vi "Main Tclk.vi"() -> ()   [LabVIEW 2018] (continued)
  T7 = cluster{"SEM Scan Parameters":cluster{"X size (um)":sgl, "Y size (um)":sgl, "X center (um)":dbl, "Y center (um)":dbl, "X size (V)":dbl, "X size auto":bool, "X stig":sgl[][], "Y stig":sgl[][], "X aln":sgl[][], "Y aln":sgl[][], "Scan rate (Hz)":u32, "Oversampling":u32, "Oversampling auto":bool, "Frame line rampdown ratio":sgl, "Pixel size (nm)":sgl, "WD (mm)":sgl[][], "X tiles":u8, "Y tiles":u8, "Overlap (um)":sgl, "Interlaced":bool, "dX (um)":sgl[], "dY (um)":sgl[], "Frames":u8}, "Detector Information":cluster{"Brightness A":dbl, "Contrast A":dbl, "Detector B name":string, "Brightness B":dbl, "Contrast B":dbl, "Detector C name":string, "Detector D name":string}, "SEM Options":cluster{"GetInfo":bool, "Set Det A para":bool, "Set WD":bool, "Set Mag":bool, "Set stig":bool, "Set aln":bool, "Display":bool, "Save":bool, "8-bit":bool, "Detector A":bool, "Detector B":bool, "Detector C":bool, "Detector D":bool, "Inverse A":bool, "Inverse B":bool, "Inverse C":bool, "Inverse D":bool, "Inverse PNG":bool, "Freeze":bool, "PNG only":bool, "Upload":bool, "Delete after upload":bool}, "Focus Index Options":cluster{"Keep aspect ratio":bool, "Show Focus Index":bool, "Focus Index primary grid center":bool, "X Grids":u8[][], "Y Grids":u8[][], "Primary X index":u8[][], "Primary Y index":u8[][]}, "Image fit to":u8, "File Information":cluster{"File path":path, "Notes":string, "Save recipe":bool, "Load recipe":bool, "Sample ID":string}, "Low mag SEM":cluster{"Low mag scan":bool, "Prior to main scan":bool, "Low mag interval":u32, "Low mag scan FOV (micron)":dbl, "Low mag scan rate (Hz)":u32, "Show HM box":bool}, "Mid Mag SEM":cluster{"Mid mag scan":bool, "Prior to main scan":bool, "Mid mag interval":u32, "X size (um)":sgl, "Y size (um)":sgl, "X center (um)":dbl, "Y center (um)":dbl, "Mid mag scan rate (Hz)":u32, "Pixel size (nm)":dbl, "Show MM box":bool}, "FIB-SEM Angle":dbl, "Milling para":cluster{"X resolution":u32, "Z resolution":u32, "X offset (um)":sgl, "Z offset (um)":sgl, "X center (um)":sgl, "Z center (um)":sgl, "X size (um)":sgl, "Z size (um)":sgl, "UL-Ang":sgl, "UR-Ang":sgl, "Line milling time (s)":sgl, "Z-step (nm)":dbl, "Lines auto pause":u16, "Auto pause":bool, "Mill from Bottom":bool, "FIB FOV (um)":sgl, "Auto Profile":bool, "Mill start from Last":bool, "FIB PID on":bool, "FIB PID reset":bool, "FIB PID measured":u8, "FIB PID target":sgl, "FIB PID target slope":sgl, "FIB PID P":sgl, "FIB PID I":sgl, "FIB PID D":sgl, "Emission (uA)":dbl, "Suppressor (V)":sgl, "Auto reheat":bool}, "FI Detector":u16, "Auto Optimzation":bool, "Images per Auto Optimization":u16, "AF Range (nm)":dbl, "AF Steps":u8, "AS Range (%)":dbl, "AS Steps":u8, "AA Range (%)":sgl, "AA Steps":u8, "X shift (nm/frame)":dbl, "Y shift (nm/frame)":dbl, "FIB Y zoom pixel (nm)":dbl, "Mail server":string, "Email Alert Recipents":string[], "Alert Settings":cluster{"3D imaging paused alarm":bool, "FIB emission limit warning":bool, "Low limit":sgl, "High limit":sgl, "Specimen @ SEM alarm":bool, "FIB CL current alarm":bool, "Beam Dump 1 alarm":bool, "Milling Z voltage alarm":bool, "EHT off alarm":bool, "Detector over scale warning":bool, "Image clipping alarm":bool, "Warning limit (um)":sgl, "Stop limit (um)":sgl, "Temperature alarm":bool, "Pause 3D-ING":bool, "Low limit (F)":sgl, "High limit (F)":sgl, "Temp limit auto":bool, "Delta (F)":sgl, "Gradient limit (F/min)":sgl, "SW error warning":bool, "Focus index warning":bool, "Focus index low limit":sgl, "Focus index stop limit":sgl, "Run Auto Stig":bool, "FI low limit auto":bool, "FI stop limit auto":bool}, "Reheat Parameters":cluster{"Filament I (A)":sgl, "Reheat time (s)":sgl, "Emission (uA)":sgl, "Calculate V/I slope":bool, "Pre-calc delay (min)":sgl, "Disable Reheat Retries":bool, "Restore Voltages":bool}, "Start FIB HV DataLog":bool, "Interval (s)":u16}
  T8 = cluster{"Brightness A":dbl, "Contrast A":dbl, "Detector B name":string, "Brightness B":dbl, "Contrast B":dbl, "Detector C name":string, "Detector D name":string}
  T9 = cluster{"SEM X coil":refnum<k15>, "SEM Y coil":refnum<k15>, "Detectors A&B":refnum<k15>, "Det min (V)":dbl, "Det max (V)":dbl, "Eanable COM":bool, "COM port":refnum<visa-resource-name>, "Detector FIB-NI auto switch":tag, "Machine Type":u8, "Machine ID":string}
  T10 = enum16{"SEM", "FIB", "Milling", "SEM + FIB", "Mill + SEM", "SEM Drift Correction", "FIB Drift Correction", "No Beam", "External", "External + SEM"}
  T11 = enum32{"Status", "Throughput", "SEM", "HV Data", "FIB", "Re-engage"}
  T12 = cluster{"AO SampClk.MaxRate":dbl, "AI SampClk.MaxRate":dbl, "AO rate":dbl, "Scan speed":u8, "Detector #":u8, "X min (V)":dbl, "X max (V)":dbl, "X min index":i32, "X max index":i32, "AO multiline":u32, "Decimating factor":u16, "AvailSampPerChan":u32, "AO scan line":u32, "Total pixels recorded":i32, "Lines scanned":i32, "Scan time (m)":dbl, "Scan time (s)":dbl, "Remaining time (m)":u16, "Remaining time (s)":u8, "SEM Spec. I (nA)":sgl, "Frame":u8, "X tile":u8, "Y tile":u8}
  T13 = cluster{"Detector A":string, "Detector B":string, "Brightness A":sgl, "Contrast A":sgl, "Brightness B":sgl, "Contrast B":sgl, "Magnification":sgl, "Pixel size":sgl, "Working distance":sgl, "EHT":sgl, "Aperture":u8, "High current mode":u8, "Probe current":sgl, "Scan rotation":sgl, "Chamber vac":sgl, "Gun vac":sgl, "Beam shift X":sgl, "Beam shift Y":sgl, "Stig X":sgl, "Stig Y":sgl, "Alignment X":sgl, "Alignment Y":sgl, "Stage X":sgl, "Stage Y":sgl, "Stage Z":sgl, "Stage T":sgl, "Stage R":sgl, "Stage M":sgl}
  T14 = cluster{"A Img Focus Index":sgl, "B Img Focus Index":sgl, "C Img Focus Index":sgl, "D Img Focus Index":sgl}
  T15 = cluster{"A Img Focus Index array":dbl[][], "B Img Focus Index array":dbl[][], "C Img Focux Index array":dbl[][], "D Img Focus Index array":dbl[][]}
  T16 = cluster{"Ext Target (V)":sgl, "Ext Actual (V)":sgl, "Fil Age (hr)":sgl, "Ext I Actual (uA)":sgl, "Fil I Target (A)":sgl, "Fil I Actual (A)":sgl, "Liner Target (V)":sgl, "Liner Actual (V)":sgl, "EHT Target (V)":sgl, "EHT Actual (V)":sgl, "Supp Actual (V)":sgl, "Supp Monitor (V)":sgl, "Gun Vac (Torr)":sgl, "Sys Vac (Torr)":sgl}
  T17 = cluster{"Filament (A)":sgl, "Accelerator Target (V)":sgl, "Accelerator Actual (V)":sgl, "Extrator Target (V)":sgl, "Extrator Actual (V)":sgl, "Emission Target (uA)":sgl, "Emission Actual (uA)":sgl, "Suppressor (V)":sgl, "Faraday I (nA)":sgl, "Lens1 Target (V)":sgl, "Lens1 Actual (V)":sgl, "Lens2 Target (V)":sgl, "Lens2 Actual (V)":sgl, "Gun Vac (Torr)":sgl, "Column Vac (Torr)":sgl, "Tip Lifetime (uAhr)":sgl}
  T18 = cluster{"Filament (A)":sgl, "Accelerator (V)":sgl, "AccI (uA)":sgl, "Extrator (V)":sgl, "Emission (uA)":sgl, "Suppressor (V)":sgl, "SuppI (uA)":sgl, "Lens1 (V)":sgl, "Lens1I (uA)":sgl, "Lens2 (V)":sgl, "Lens2I (uA)":sgl, "Tip Lifetime (hr)":sgl}
  T19 = cluster{"FIB mode":u8, "FIB focus":sgl, "FIB probe current":sgl, "FIB emission (uA)":sgl, "FIB rotation":sgl, "FIB aperture X":sgl, "FIB aperture Y":sgl, "FIB stig X":sgl, "FIB stig Y":sgl, "FIB beam shift X":sgl, "FIB beam shift Y":sgl}
  T20 = cluster{"Actual scan rate":dbl, "X resolution with rampdown":i32, "Actual sample rate":dbl, "Fetch backlog":dbl, "Total scan points":i32, "Frame rate (/s)":u32}
  T21 = cluster{"Reheat finish time":string, "Reheat Success":bool, "Initial emission (uA)":sgl, "Initial suppressor (V)":sgl, "V/I Slope":sgl}
  T22 = typedef "LVPoint32TypeDef.ctl" = cluster{"Horizontal":i32, "Vertical":i32}
  T23 = cluster{"FIB X coil":tag, "FIB Y coil":tag, "Beam blank":tag, "FIB Ext Scan":tag, "Detector":tag, "Post #1up":tag, "Post #1down":tag, "Post #2up":tag, "Post #2down":tag}
  T24 = enum32{"Hardware", "SEM", "Add'l SEM's", "File & Logging", "FIB Imaging", "FIB Reheat", "FIB Milling", "Alert"}
  T25 = cluster{"SEM X coil":refnum<k15>, "SEM Y coil":refnum<k15>, "FIB X coil":tag, "FIB Y coil":tag, "FIB Detector":tag, "SEM Detectors":refnum<k15>, "Det min (V)":dbl, "Det max (V)":dbl, "Eanable COM":bool, "COM port":refnum<visa-resource-name>, "FIB Beam blank":tag, "FIB Ext Scan":tag, "Det. FIB-NI auto switch":tag, "Post #1up":tag, "Post #1down":tag, "Post #2up":tag, "Post #2down":tag, "Machine Type":u8, "FIB Faraday Cup":tag, "Configuration file":path, "SEM Max FOV (um)":sgl, "Machine ID":string, "Save config file":bool, "Temperature port":refnum<visa-resource-name>, "Brightness A":dbl, "Contrast A":dbl, "Detector B name":string, "Brightness B":dbl, "Contrast B":dbl, "Logging Device":tag}
  T26 = cluster{"X size (um)":sgl, "Y size (um)":sgl, "X center (um)":sgl, "Y center (um)":sgl, "X size (V)":dbl, "X size auto":bool, "X stig":sgl[][], "Y stig":sgl[][], "X aln":sgl[][], "Y aln":sgl[][], "Scan rate (Hz)":u32, "Oversampling":u32, "Oversampling auto":bool, "Frame line rampdown ratio":sgl, "Pixel size (nm)":sgl, "WD (mm)":sgl[][], "X tiles":u8, "Y tiles":u8, "Overlap (um)":sgl, "Interlaced":bool, "dX (um)":sgl[], "dY (um)":sgl[], "Frames":u8}
  T27 = cluster{"GetInfo":bool, "Set Det A para":bool, "Set WD":bool, "Set Mag":bool, "Set stig":bool, "Set aln":bool, "Display":bool, "Save":bool, "8-bit":bool, "Detector A":bool, "Detector B":bool, "Detector C":bool, "Detector D":bool, "Inverse A":bool, "Inverse B":bool, "Inverse C":bool, "Inverse D":bool, "Inverse PNG":bool, "Freeze":bool, "PNG only":bool, "Upload":bool, "Delete after upload":bool}
  T28 = cluster{"Keep aspect ratio":bool, "Show Focus Index":bool, "Focus Index primary grid center":bool, "X Grids":u8[][], "Y Grids":u8[][], "Primary X index":u8[][], "Primary Y index":u8[][]}
  T29 = cluster{"Mid mag scan":bool, "Prior to main scan":bool, "Mid mag interval":u32, "X size (um)":sgl, "Y size (um)":sgl, "X center (um)":dbl, "Y center (um)":dbl, "Mid mag scan rate (Hz)":u32, "Pixel size (nm)":sgl, "Show MM box":bool}
  T30 = cluster{"Low mag scan":bool, "Prior to main scan":bool, "Low mag interval":u32, "Low mag scan FOV (micron)":dbl, "Low mag scan rate (Hz)":u32, "Show HM box":bool}
  T31 = cluster{"File path":path, "Notes":string, "Save recipe":bool, "Load recipe":bool, "Sample ID":string}
  T32 = cluster{"X resolution":u32, "Z resolution":u32, "X center":dbl, "Z center":dbl, "X size (V)":dbl, "Z size (V)":dbl, "Frame line rampdown ratio":dbl, "Scan rate (Hz)":u32, "Oversampling":u16}
  T33 = cluster{"Scan mode":u16, "Flip x":bool, "Flip z":bool, "Det":u16}
  T34 = cluster{"X resolution":u32, "Y resolution":u32, "X center":dbl, "Y center":dbl, "X size (V)":dbl, "Y size (V)":dbl, "Frame line rampdown ratio":dbl, "Scan rate (Hz)":u32, "Oversampling":u16}
  T35 = cluster{"X resolution":u32, "Z resolution":u32, "X offset (um)":sgl, "Z offset (um)":sgl, "X center (um)":sgl, "Z center (um)":sgl, "X size (um)":sgl, "Z size (um)":sgl, "UL-Ang":sgl, "UR-Ang":sgl, "Line milling time (s)":sgl, "Z-step (nm)":dbl, "Lines auto pause":u16, "Auto pause":bool, "Mill from Bottom":bool, "FIB FOV (um)":sgl, "Auto Profile":bool, "Mill start from Last":bool, "FIB PID on":bool, "FIB PID reset":bool, "FIB PID measured":u8, "FIB PID target":sgl, "FIB PID target slope":sgl, "FIB PID P":sgl, "FIB PID I":sgl, "FIB PID D":sgl, "Emission (uA)":dbl, "Suppressor (V)":sgl, "Auto reheat":bool}
  T36 = cluster{"3D imaging paused alarm":bool, "FIB emission warning":bool, "Low limit":dbl, "High limit":dbl, "Specimen @ SEM alarm":bool, "FIB CL current alarm":bool, "Beam Dump 1 alarm":bool, "Milling Z voltage alarm":bool, "EHT off alarm":bool, "Detector over scale warning":bool, "Image clipping alarm":bool, "Warning limit (um)":sgl, "Stop limit (um)":sgl, "Temperature alarm":bool, "Pause 3D-ING":bool, "Low limit (F)":sgl, "High limit (F)":sgl, "Temp limit auto":bool, "Delta (F)":sgl, "Gradient limit (F/min)":sgl, "SW error warning":bool, "Focus index warning":bool, "Focus index low limit":sgl, "Focus index stop limit":sgl, "Run Auto Stig":bool, "FI low limit auto":bool, "FI stop limit auto":bool}
  T37 = enum32{"All", "Detector A", "Detector B", "Detector A Low Mag", "Detector B Low Mag", "FIB", "FIB Milling Offset after Pause", "Auto Focus / Stig / Align", "Imaging Quality", "Temp. and Currents", "FIB HV Data", "Logging: Realtime Graphs"}
  T38 = cluster{cluster{"element":dbl, "A Img Focus Index":dbl}[]}[]
  T39 = cluster{"Log time array":u32[], "Delta X stop limit array":sgl[]}[]
  T40 = cluster{"Log time array":u32[], "Milling Y voltage array":sgl[]}
  T41 = cluster{"Log time array":u32[], "Delta Y stop limit array":sgl[]}[]
  T42 = cluster{sgl[][], sgl[][], sgl[][], sgl[][], sgl[][], sgl[], sgl[]}
  T43 = enum32{"Hardware", "SEM", "Add'l SEM's", "Data Logging", "FIB Imaging", "FIB Reheat", "FIB Milling", "Alert"}
  T44 = enum8{"Enabled", "Disabled", "Disabled and Grayed Out"}
  T45 = enum32{"Page Enabled", "Page Disabled", "Page Disabled & Grayed"}
  T46 = cluster{"left":i16, "top":i16, "right":i16, "bottom":i16}
  T47 = cluster{"Timestamp":timestamp, "Double":sgl, "FIB slice #":u32, "Reheat":bool, "Double 2":sgl, "Double 3":sgl, "Double 4":sgl}
  T48 = typedef "eventvkey.ctl" = enum16{"ASCII", "Enter", "Return", "Shift", "Ctrl", "Alt", "Cmd", "Opt", "Caps", "NumLock", "Clear", "Break", "Up", "Down", "Left", "Right", "Insert", "Delete", "Home", "End", "PageUp", "PageDown", "Escape", "Help", "Pause", "ScrollLock", "F1", "F2", "F3", "F4", "F5", "F6", "F7", "F8", "F9", "F10", "F11", "F12", "F13", "F14", "F15", "F16", "F17", "F18", "F19", "F20", "F21", "F22", "F23", "F24", "Play", "VolumeUp", "VolumeDown", "Mute", "Two Byte Char"}
  T49 = enum16{"open", "replace", "create", "open or create", "replace or create", "replace or create with confirmation"}
  T50 = enum16{"SEM", "FIB", "Mill", "SEM + FIB", "Mill + SEM", "Drift SEM", "Drift FIB", "None", "Ext", "Ext + SEM"}
  T51 = enum16{"Pages and Rows", "Pages and Columns", "Rows and Columns"}
  T52 = cluster{"A Img Focus Index":sgl[][], "B Img Focus Index":sgl[][], "C Img Focus Index":sgl[][], "D Img Focus Index":sgl[][]}
  T53 = cluster{"A Img Focus Index array":sgl[][][][], "B Img Focus Index array":sgl[][][][], "C Img Focus Index array":sgl[][][][], "D Img Focus Index array":sgl[][][][]}
  T54 = cluster{"SEM Status":cluster{"AO SampClk.MaxRate":dbl, "AI SampClk.MaxRate":dbl, "AO rate":dbl, "Scan speed":u8, "Detector #":u8, "X min (V)":dbl, "X max (V)":dbl, "X min index":i32, "X max index":i32, "AO multiline":u32, "Decimating factor":u16, "AvailSampPerChan":u32, "AO scan line":u32, "Total pixels recorded":i32, "Lines scanned":i32, "Scan time (m)":dbl, "Scan time (s)":dbl, "Remaining time (m)":u16, "Remaining time (s)":u8, "SEM Spec. I (nA)":sgl, "Frame":u8, "X tile":u8, "Y tile":u8}, "SEM Parameters":cluster{"Detector A":string, "Detector B":string, "Brightness A":sgl, "Contrast A":sgl, "Brightness B":sgl, "Contrast B":sgl, "Magnification":sgl, "Pixel size":sgl, "Working distance":sgl, "EHT":sgl, "Aperture":u8, "High current mode":u8, "Probe current":sgl, "Scan rotation":sgl, "Chamber vac":sgl, "Gun vac":sgl, "Beam shift X":sgl, "Beam shift Y":sgl, "Stig X":sgl, "Stig Y":sgl, "Alignment X":sgl, "Alignment Y":sgl, "Stage X":sgl, "Stage Y":sgl, "Stage Z":sgl, "Stage T":sgl, "Stage R":sgl, "Stage M":sgl}, "Image Focus Index":cluster{"A Img Focus Index":sgl, "B Img Focus Index":sgl, "C Img Focus Index":sgl, "D Img Focus Index":sgl}, "FIB parameters":cluster{"FIB mode":u8, "FIB focus":sgl, "FIB probe current":sgl, "FIB emission current":sgl, "FIB rotation":sgl, "FIB aperture X":sgl, "FIB aperture Y":sgl, "FIB stig X":sgl, "FIB stig Y":sgl, "FIB beam shift X":sgl, "FIB beam shift Y":sgl}, "Image Focus Index Array":cluster{"A Img Focus Index array":sgl[][], "B Img Focus Index array":sgl[][], "C Img Focus Index array":sgl[][], "D Img Focus Index array":sgl[][]}}
  T55 = typedef "imagedata.ctl" = cluster{"image type":i32, "image depth":i32, "image":u8[], "mask":u8[], "colors":u32[], "Rectangle":cluster{"left":i16, "top":i16, "right":i16, "bottom":i16}}
  T56 = cluster{"FIB mode":u8, "FIB focus":sgl, "FIB probe current":sgl, "FIB emission current":sgl, "FIB rotation":sgl, "FIB aperture X":sgl, "FIB aperture Y":sgl, "FIB stig X":sgl, "FIB stig Y":sgl, "FIB beam shift X":sgl, "FIB beam shift Y":sgl}
  T57 = cluster{"Timestamp":timestamp, "Milling Z voltage (V)":sgl, "FIB slice #":u32, "Pause for reheat":bool, "Last good FI":sgl, "Focus Index":sgl, "SEM Max FOV (um)":sgl}
  T58 = cluster{u32[], "Faraday Cup high limit array":sgl[]}
  T59 = cluster{u32[], "Faraday Cup low limit array":sgl[]}
  T60 = cluster{u32[], "SEM Specimen I high limit array":sgl[]}
  T61 = cluster{u32[], "Specimen I high limit array":sgl[]}
  T62 = cluster{u32[], "Specimen I low limit array":sgl[]}
  T63 = cluster{u32[], "SEM Specimen I low limit array":sgl[]}
  T64 = cluster{u32[], "Milling I high limit array":sgl[]}
  T65 = cluster{u32[], "Milling I low limit array":sgl[]}
  T66 = cluster{u32[], "Faraday Cup low limit array":sgl[]}[]
  T67 = cluster{u32[], "Specimen I low limit array":sgl[]}[]
  T68 = cluster{u32[], "SEM Specimen I low limit array":sgl[]}[]
  T69 = cluster{u32[], "Milling I low limit array":sgl[]}[]
  T70 = typedef "LVRangeTypeDef.ctl" = cluster{"Minimum":dbl, "Maximum":dbl, "Increment":dbl, "Minor Increment":dbl, "Start":dbl}
  T71 = typedef "LVRectTypeDef.ctl" = cluster{"Left":i16, "Top":i16, "Right":i16, "Bottom":i16}
  T72 = cluster{u32[], "Delta X stop limit array":sgl[]}[]
  T73 = cluster{u32[], "Delta Y stop limit array":sgl[]}[]
  T74 = cluster{cluster{"Center":sgl, "A Img Focus Index":sgl}[]}
  T75 = cluster{cluster{"Center":sgl, "A Img Focus Index":sgl}[]}[]
  T76 = cluster{cluster{"Center":dbl, "A Img Focus Index":dbl}[]}[]
  T77 = cluster{"Shift":bool, "Ctrl":bool, "Alt":bool, "Cmd":bool, "Opt":bool}
  T78 = enum16{"Left Button", "Center Button", "Right Button", "Window Close"}
  T79 = cluster{"AI sampling time increment":dbl, "AI scaling coefficients":sgl[][], "AI channels":cluster{"AI 1":bool, "AI 2":bool, "AI 3":bool, "AI 4":bool}, "Resolution and scan":cluster{"X resolution":u32, "Z resolution":u32, "AI oversampling":u16, "Scan speed":u8, "Actual AO rate":dbl, "Frame line rampdown ratio":dbl, "X min (V)":dbl, "X max (V)":dbl, "Det min (V)":dbl, "Det max (V)":dbl}, "Decimating factor":u16, "Notes":string, "Other detectors":cluster{"Detector C name":string, "Detector D name":string}, "SEM parameters":cluster{"Detector A":string, "Detector B":string, "Brightness A":sgl, "Contrast A":sgl, "Brightness B":sgl, "Contrast B":sgl, "Magnification":sgl, "Pixel size":sgl, "Working distance":sgl, "EHT":sgl, "Aperture":u8, "High current mode":u8, "Probe current":sgl, "Scan rotation":sgl, "Chamber vac":sgl, "Gun vac":sgl, "Beam shift X":sgl, "Beam shift Y":sgl, "Stig X":sgl, "Stig Y":sgl, "Alignment X":sgl, "Alignment Y":sgl, "Stage X":sgl, "Stage Y":sgl, "Stage Z":sgl, "Stage T":sgl, "Stage R":sgl, "Stage M":sgl}, "FIB parameters":cluster{"FIB mode":u8, "FIB focus":sgl, "FIB probe current":u8, "FIB emission current":sgl, "FIB rotation":sgl, "FIB aperture X":sgl, "FIB aperture Y":sgl, "FIB stig X":sgl, "FIB stig Y":sgl, "FIB beam shift X":sgl, "FIB beam shift Y":sgl}, "Milling para":cluster{"X resolution":u32, "Z resolution":u32, "X offset (um)":sgl, "Z offset (um)":sgl, "X center (um)":sgl, "Z center (um)":sgl, "X size (um)":sgl, "Z size (um)":sgl, "UL-Ang":sgl, "UR-Ang":sgl, "Line milling time (s)":sgl, "Z-step (nm)":dbl, "Lines auto pause":u16, "Auto pause":bool, "Mill from Bottom":bool, "FIB FOV (um)":sgl, "Auto Profile":bool, "Mill start from Last":bool, "FIB PID on":bool, "FIB PID reset":bool, "FIB PID measured":u8, "FIB PID target":sgl, "FIB PID target slope":sgl, "FIB PID P":sgl, "FIB PID I":sgl, "FIB PID D":sgl, "Emission (uA)":dbl, "Suppressor (V)":sgl, "Auto reheat":bool}, "Machine ID":string, "Data Logging":cluster{"Temp (F)":sgl, "FIB Faraday Cup (nA)":sgl, "FIB Specimen I (nA)":sgl, "Beam Dump 1 (nA)":sgl, "Beam Dump 2 (nA)":sgl, "Milling I (nA)":sgl, "SEM Specimen I (nA)":sgl, "Milling Z voltage (V)":sgl, "Focus Index":sgl, "FIB slice #":u32}}
  T80 = cluster{"FIB mode":u8, "FIB focus":sgl, "FIB probe current":u8, "FIB emission current":sgl, "FIB rotation":sgl, "FIB aperture X":sgl, "FIB aperture Y":sgl, "FIB stig X":sgl, "FIB stig Y":sgl, "FIB beam shift X":sgl, "FIB beam shift Y":sgl}
  T81 = cluster{"Temp (F)":sgl, "FIB Faraday Cup (nA)":sgl, "FIB Specimen I (nA)":sgl, "Beam Dump 1 (nA)":sgl, "Beam Dump 2 (nA)":sgl, "Milling I (nA)":sgl, "SEM Specimen I (nA)":sgl, "Milling Z voltage (V)":sgl, "Focus Index":sgl, "FIB slice #":u32}
  T82 = typedef "DialogType.ctl" = u16
  T83 = cluster{"Log time array":u32[], "Delta X array":sgl[]}
  T84 = cluster{"Log time array":u32[], "Delta X stop limit array":sgl[]}
  T85 = cluster{"Log time array":u32[], "Delta X sum array":sgl[]}
  T86 = cluster{"Log time array":u32[], "Delta X sum array":sgl[]}[]
  T87 = cluster{"Log time array":u32[], "Delta Y array":sgl[]}
  T88 = cluster{"Log time array":u32[], "Delta Y sum array":sgl[]}
  T89 = cluster{"Log time array":u32[], "Delta Y sum array":sgl[]}[]
  T90 = cluster{"Log time array":u32[], "Delta Z array":sgl[]}
  T91 = cluster{"Log time array":u32[], "Milling Z voltage array":sgl[]}
  T92 = cluster{"Log time array":u32[], "Delta image array":sgl[]}
  T93 = cluster{"Log time array":u32[], "Specimen I array":sgl[]}
  T94 = cluster{"Log time array":u32[], "Specimen I high limit array":sgl[]}
  T95 = cluster{"Log time array":u32[], "Specimen I low limit array":sgl[]}
  T96 = cluster{"Log time array":u32[], "Specimen I low limit array":sgl[]}[]
  T97 = cluster{"Log time array":u32[], "SEM Specimen I array":sgl[]}
  T98 = cluster{"Log time array":u32[], "SEM Specimen I high limit array":sgl[]}
  T99 = cluster{"Log time array":u32[], "SEM Specimen I low limit array":sgl[]}
  T100 = cluster{"Log time array":u32[], "SEM Specimen I low limit array":sgl[]}[]
  T101 = cluster{"Log time array":u32[], "Beam Dump 2 array":sgl[]}
  T102 = cluster{"Log time array":u32[], "BD2 high limit array":sgl[]}
  T103 = cluster{"Log time array":u32[], "BD2 low limit array":sgl[]}
  T104 = cluster{"Log time array":u32[], "BD2 low limit array":sgl[]}[]
  T105 = cluster{"Log time array":u32[], "Milling I array":sgl[]}
  T106 = cluster{"Log time array":u32[], "Milling I high limit array":sgl[]}
  T107 = cluster{"Log time array":u32[], "Milling I low limit array":sgl[]}
  T108 = cluster{"Log time array":u32[], "Milling I low limit array":sgl[]}[]
  T109 = cluster{"Log time array":u32[], "Beam Dump 1 array":sgl[]}
  T110 = cluster{"Log time array":u32[], "BD1 high limit array":sgl[]}
  T111 = cluster{"Log time array":u32[], "BD1 low limit array":sgl[]}
  T112 = cluster{"Log time array":u32[], "BD1 low limit array":sgl[]}[]
  T113 = cluster{"Filament (A)":sgl, "Acclerator (V)":sgl, "AccI (uA)":sgl, "Extractor (V)":sgl, "Emission (uA)":sgl, "Suppressor (V)":sgl, "SuppI (uA)":sgl, "Lens1 (V)":sgl, "Lens1I (uA)":sgl, "Lens2 (V)":sgl, "Lens2I (uA)":sgl, "Tip Lifetime (hr)":sgl}
  T114 = cluster{"SEM Scan Parameters":cluster{"X size (um)":sgl, "Y size (um)":sgl, "X center (um)":dbl, "Y center (um)":dbl, "X size (V)":dbl, "X size auto":bool, "X stig":sgl[][], "Y stig":sgl[][], "X aln":sgl[][], "Y aln":sgl[][], "Scan rate (Hz)":u32, "Oversampling":u32, "Oversampling auto":bool, "Frame line rampdown ratio":sgl, "Pixel size (nm)":sgl, "WD (mm)":sgl[][], "X tiles":u8, "Y tiles":u8, "Overlap (um)":sgl, "Interlaced":bool, "dX (um)":sgl[], "dY (um)":sgl[], "Frames":u8}, "Detector Information":cluster{"Brightness A":dbl, "Contrast A":dbl, "Detector B name":string, "Brightness B":dbl, "Contrast B":dbl, "Detector C name":string, "Detector D name":string}, "SEM Options":cluster{"GetInfo":bool, "Set Det A para":bool, "Set WD":bool, "Set Mag":bool, "Set stig":bool, "Set aln":bool, "Display":bool, "Save":bool, "8-bit":bool, "Detector A":bool, "Detector B":bool, "Detector C":bool, "Detector D":bool, "Inverse A":bool, "Inverse B":bool, "Inverse C":bool, "Inverse D":bool, "Inverse PNG":bool, "Freeze":bool, "PNG only":bool, "Upload":bool, "Delete after upload":bool}, "Focus Index Options":cluster{"Keep aspect ratio":bool, "Show Focus Index":bool, "Focus Index primary grid center":bool, "X Grids":u8[][], "Y Grids":u8[][], "Primary X index":u8[][], "Primary Y index":u8[][]}, "Image fit to":u8, "File Information":cluster{"File path":path, "Notes":string, "Save recipe":bool, "Load recipe":bool, "Sample ID":string}, "Low mag SEM":cluster{"Low mag scan":bool, "Prior to main scan":bool, "Low mag interval":u32, "Low mag scan FOV (micron)":dbl, "Low mag scan rate (Hz)":u32, "Show HM box":bool}, "Mid Mag SEM":cluster{"Mid mag scan":bool, "Prior to main scan":bool, "Mid mag interval":u32, "X size (um)":sgl, "Y size (um)":sgl, "X center (um)":dbl, "Y center (um)":dbl, "Mid mag scan rate (Hz)":u32, "Pixel size (nm)":dbl, "Show MM box":bool}, "FIB-SEM Angle":dbl, "Milling para":cluster{"X resolution":u32, "Z resolution":u32, "X offset (um)":sgl, "Z offset (um)":sgl, "X center (um)":sgl, "Z center (um)":sgl, "X size (um)":sgl, "Z size (um)":sgl, "UL-Ang":sgl, "UR-Ang":sgl, "Line milling time (s)":sgl, "Z-step (nm)":dbl, "Lines auto pause":u16, "Auto pause":bool, "Mill from Bottom":bool, "FIB FOV (um)":sgl, "Auto Profile":bool, "Mill start from Last":bool, "FIB PID on":bool, "FIB PID reset":bool, "FIB PID measured":u8, "FIB PID target":sgl, "FIB PID target slope":sgl, "FIB PID P":sgl, "FIB PID I":sgl, "FIB PID D":sgl, "Emission (uA)":dbl, "Suppressor (V)":sgl, "Auto reheat":bool}, "FI Detector":u16, "Auto Optimzation":bool, "Images per Auto Optimization":u16, "AF Range (nm)":sgl, "AF Steps":u8, "AS Range (%)":sgl, "AS Steps":u8, "AA Range (%)":sgl, "AA Steps":u8, "X shift (nm/frame)":dbl, "Y shift (nm/frame)":dbl, "FIB Y zoom pixel (nm)":dbl, "Mail server":string, "Email Alert Recipients":string[], "Alert Settings":cluster{"3D imaging paused alarm":bool, "FIB emission limit warning":bool, "Low limit":sgl, "High limit":sgl, "Specimen @ SEM alarm":bool, "FIB CL current alarm":bool, "Beam Dump 1 alarm":bool, "Milling Z voltage alarm":bool, "EHT off alarm":bool, "Detector over scale warning":bool, "Image clipping alarm":bool, "Warning limit (um)":sgl, "Stop limit (um)":sgl, "Temperature alarm":bool, "Pause 3D-ING":bool, "Low limit (F)":sgl, "High limit (F)":sgl, "Temp limit auto":bool, "Delta (F)":sgl, "Gradient limit (F/min)":sgl, "SW error warning":bool, "Focus index warning":bool, "Focus index low limit":sgl, "Focus index stop limit":sgl, "Run Auto Stig":bool, "FI low limit auto":bool, "FI stop limit auto":bool}, "Reheat Parameters":cluster{"Filament I (A)":sgl, "Reheat time (s)":sgl, "Emission (uA)":sgl, "Calculate V/I slope":bool, "Pre-calc delay (min)":sgl, "Disable Reheat Retries":bool, "Restore Voltages":bool}, "Start FIB HV DataLog":bool, "Interval (s)":u16}
  T115 = cluster{"Mid mag scan":bool, "Prior to main scan":bool, "Mid mag interval":u32, "X size (um)":sgl, "Y size (um)":sgl, "X center (um)":dbl, "Y center (um)":dbl, "Mid mag scan rate (Hz)":u32, "Pixel size (nm)":dbl, "Show MM box":bool}
  T116 = cluster{"3D imaging paused alarm":bool, "FIB emission limit warning":bool, "Low limit":sgl, "High limit":sgl, "Specimen @ SEM alarm":bool, "FIB CL current alarm":bool, "Beam Dump 1 alarm":bool, "Milling Z voltage alarm":bool, "EHT off alarm":bool, "Detector over scale warning":bool, "Image clipping alarm":bool, "Warning limit (um)":sgl, "Stop limit (um)":sgl, "Temperature alarm":bool, "Pause 3D-ING":bool, "Low limit (F)":sgl, "High limit (F)":sgl, "Temp limit auto":bool, "Delta (F)":sgl, "Gradient limit (F/min)":sgl, "SW error warning":bool, "Focus index warning":bool, "Focus index low limit":sgl, "Focus index stop limit":sgl, "Run Auto Stig":bool, "FI low limit auto":bool, "FI stop limit auto":bool}
  T117 = cluster{"Suppressor (V)":sgl, "Emission (uA)":sgl}
  T118 = cluster{"Suppressor (V)":sgl, "Emission Actual (uA)":sgl}
diagram:
  n1 = local read "SEM Scan Parameters"() -> (w7:T26)
  n2 = Unbundle By Name(w7) -> ("X stig"=w1:sgl[][], "Y stig"=w2:sgl[][], "X aln"=w3:sgl[][], "Y aln"=w4:sgl[][], "WD (mm)"=w5:sgl[][])
  n3 = Build Array(w1, w2, w3, w4, w5) -> (w6:sgl[][][])
  n4 = for {
    tunnel: w6 -> [w16] mode=indexing
    tunnel: [w19] -> w9 mode=indexing
    workers-P: _ -> [_]
    w18 = 1 ("dimension size")
    n5 = Array Size(array=w16) -> (size(s)=w17:i32[])
    n6 = Multiply Array Elements(1:w17) -> (0:w15:i32)
    n7 = Reshape Array(w16, w15) -> (w21:sgl[])
    n8 = call-poly <vilib>:"Mean.vi"("X"=w21) -> ("mean"=w20:dbl)  [unwired: 1 out]
    n9 = Initialize Array(w20, w18, w18) -> (w19:dbl[][])
  }
  n10 = Index Array(array=w9) -> (element #1=w10:dbl[][], element #2=w11:dbl[][], element #3=w12:dbl[][], element #4=w13:dbl[][], element #5=w14:dbl[][])  [unwired: 15 in]
  n11 = Bundle By Name(cluster=w7, "X stig"=w10, "Y stig"=w11, "X aln"=w12, "Y aln"=w13, "WD (mm)"=w14) -> (w8:T26)
  n12 = local write "SEM Scan Parameters"(w8) -> ()
  n13 = stacked-sequence {
    frame #0 {
      n14 = disable-structure shown="Disabled" {
        frame Disabled {
          w36 = string[] ["Machine ID", "Machine type", "SEM maximum FOV (um)", "Detector min (V)", "Detector max (V)", "Brightness A", "Contrast A", "Detector B name", "Brightness B", "Contrast B"]
          n15 = local read "Hardware Configuration"() -> (w104:T25)
          n16 = Unbundle By Name(w104) -> ("Configuration file"=w105:path)
          n17 = call-poly <vilib>:"Read From Spreadsheet File.vi"("delimiter (\\t)"="," ("delimiter (\\t)"), "file path (dialog if empty)"=w105) -> ("all rows"=w37:string[][])  [unwired: 5 in, 4 out]
          n18 = Index Array(array=w36, index=0) -> (element=w62:string)
          n19 = Index Array(array=w36, index=1) -> (element=w59:string)
          n20 = Index Array(array=w36, index=2) -> (element=w50:string)
          n21 = Index Array(array=w36, index=3) -> (element=w48:string)
          n22 = Index Array(array=w36, index=4) -> (element=w49:string)
          n23 = Index Array(array=w36, index=5) -> (element=w47:string)
          n24 = Index Array(array=w36, index=6) -> (element=w46:string)
          n25 = Index Array(array=w36, index=7) -> (element=w45:string)
          n26 = Index Array(array=w36, index=8) -> (element=w44:string)
          n27 = Index Array(array=w36, index=9) -> (element=w43:string)
          n28 = call "2D array search.vi"("Search For"=w62, "Input Array"=w37) -> ("Column"=w75:i32, "Row"=w74:i32)  [unwired: 7 in, 1 out]
          n29 = call "2D array search.vi"("Search For"=w59, "Input Array"=w37) -> ("Column"=w96:i32, "Row"=w97:i32)  [unwired: 7 in, 1 out]
          n30 = call "2D array search.vi"("Search For"=w50, "Input Array"=w37) -> ("Column"=w94:i32, "Row"=w93:i32)  [unwired: 7 in, 1 out]
          n31 = call "2D array search.vi"("Search For"=w48, "Input Array"=w37) -> ("Column"=w67:i32, "Row"=w69:i32)  [unwired: 7 in, 1 out]
          n32 = call "2D array search.vi"("Search For"=w49, "Input Array"=w37) -> ("Column"=w70:i32, "Row"=w72:i32)  [unwired: 7 in, 1 out]
          n33 = call "2D array search.vi"("Search For"=w47, "Input Array"=w37) -> ("Column"=w91:i32, "Row"=w89:i32)  [unwired: 7 in, 1 out]
          n34 = call "2D array search.vi"("Search For"=w46, "Input Array"=w37) -> ("Column"=w88:i32, "Row"=w86:i32)  [unwired: 7 in, 1 out]
          n35 = call "2D array search.vi"("Search For"=w45, "Input Array"=w37) -> ("Column"=w85:i32, "Row"=w83:i32)  [unwired: 7 in, 1 out]
          n36 = call "2D array search.vi"("Search For"=w44, "Input Array"=w37) -> ("Column"=w82:i32, "Row"=w80:i32)  [unwired: 7 in, 1 out]
          n37 = call "2D array search.vi"("Search For"=w43, "Input Array"=w37) -> ("Column"=w79:i32, "Row"=w77:i32)  [unwired: 7 in, 1 out]
          n38 = Increment(x=w75) -> (x+1=w76:i32)
          n39 = Increment(x=w96) -> (x+1=w95:i32)
          n40 = Increment(x=w94) -> (x+1=w92:i32)
          n41 = Increment(x=w67) -> (x+1=w68:i32)
          n42 = Increment(x=w70) -> (x+1=w71:i32)
          n43 = Increment(x=w91) -> (x+1=w90:i32)
          n44 = Increment(x=w88) -> (x+1=w87:i32)
          n45 = Increment(x=w85) -> (x+1=w84:i32)
          n46 = Increment(x=w82) -> (x+1=w81:i32)
          n47 = Increment(x=w79) -> (x+1=w78:i32)
          n48 = Index Array(array=w37, index (row)=w74, index (col)=w76) -> (element=w73:string)
          n49 = Index Array(array=w37, index (row)=w97, index (col)=w95) -> (element=w107:string)
          n50 = Index Array(array=w37, index (row)=w93, index (col)=w92) -> (element=w99:string)
          n51 = Index Array(array=w37, index (row)=w69, index (col)=w68) -> (element=w66:string)
          n52 = Index Array(array=w37, index (row)=w72, index (col)=w71) -> (element=w65:string)
          n53 = Index Array(array=w37, index (row)=w89, index (col)=w90) -> (element=w103:string)
          n54 = Index Array(array=w37, index (row)=w86, index (col)=w87) -> (element=w102:string)
          n55 = Index Array(array=w37, index (row)=w83, index (col)=w84) -> (element=w40:string)
          n56 = Index Array(array=w37, index (row)=w80, index (col)=w81) -> (element=w100:string)
          n57 = Index Array(array=w37, index (row)=w77, index (col)=w78) -> (element=w101:string)
          n58 = case shown="\"Feiss\", Default" w107 {
            tunnel: [u8 0 ("Machine Type") u8 2 ("Machine Type") u8 1 ("Machine Type")] -> w106
            frame "Feiss", Default {
            }
            frame "Jeiss" {
            }
            frame "NVision" {
            }
          }
          n59 = Fract/Exp String To Number(string=w99) -> (number=w98:dbl)  [unwired: 4 out]
          n60 = Fract/Exp String To Number(string=w66) -> (number=w64:dbl)  [unwired: 4 out]
          n61 = Fract/Exp String To Number(string=w65) -> (number=w63:dbl)  [unwired: 4 out]
          n62 = Fract/Exp String To Number(string=w103) -> (number=w42:dbl)  [unwired: 4 out]
          n63 = Fract/Exp String To Number(string=w102) -> (number=w41:dbl)  [unwired: 4 out]
          n64 = Fract/Exp String To Number(string=w100) -> (number=w39:dbl)  [unwired: 4 out]
          n65 = Fract/Exp String To Number(string=w101) -> (number=w38:dbl)  [unwired: 4 out]
          n66 = Bundle By Name(cluster=w104, "Machine ID"=w73, "Machine Type"=w106, "SEM Max FOV (um)"=w98, "Det min (V)"=w64, "Det max (V)"=w63, "Brightness A"=w42, "Contrast A"=w41, "Detector B name"=w40, "Brightness B"=w39, "Contrast B"=w38) -> (w108:T25)
          n67 = local write "Hardware Configuration"(w108) -> ()
          "HW config items" <- w36
        }
        frame Enabled {
        }
      }
      n68 = flat-sequence {
        frame #0 {
          n69 = local read "Hardware Configuration"() -> (w23:T25)
          n70 = shared-variable ".\\Zeiss Library.lvlib\\SW date"("SW date") -> ()  [unwired: 1 in, 1 out]
          n71 = call "Read Config Settings from INI file.vi"("Hardware Configuration"=w23) -> ("Hardware Configuration Out"=w24:T25)  [unwired: 9 in]
          n72 = local write "Hardware Configuration"(w24) -> ()
        }
        frame #1 {
          n73 = local read "SEM HW Config"() -> (w25:T9)
          n74 = local read "FIB HW Config"() -> (w33:T23)
          n75 = Unbundle By Name(w25) -> ("SEM X coil"=w26:refnum<k15>)
          n76 = Unbundle By Name(w33) -> ("FIB X coil"=w34:tag)
          n77 = Type Cast(x=w26) -> (*(type *) &x=w27:string)  [unwired: 1 in]
          n78 = Type Cast(x=w34) -> (*(type *) &x=w32:string)  [unwired: 1 in]
          n79 = Match Pattern(string=w27, regular expression="/") -> (before substring=w29:string)  [unwired: 1 in, 3 out]
          n80 = Match Pattern(string=w32, regular expression="/") -> (before substring=w30:string)  [unwired: 1 in, 3 out]
          n81 = call <vilib>:"DAQmx Reset Device.vi"("device in"=w29) -> ()  [unwired: 14 in, 1 out]
          n82 = call <vilib>:"DAQmx Reset Device.vi"("device in"=w30) -> ()  [unwired: 14 in, 1 out]
        }
        frame #2 {
          n83 = shared-variable ".\\Zeiss Library.lvlib\\Force tclk init"(TRUE ("Force tclk init")) -> ()  [unwired: 1 in, 1 out]
        }
      }
    }
    frame #1 {
      w191 = sgl[][] [] ("FI array")
      w193 = bool[][] [[FALSE]] ("AF Success tiled")
      w240 = FALSE ("Visible")
      w129 = path "D:/3D FIB-SEM Files" ("path")
      w189 = sgl[][][] [] ("FI grid array")
      w149 = u32[] [] ("FI array")
      w119 = sgl 20.0 ("t")
      w217 = T44."Disabled and Grayed Out" ("Disabled")
      w125 = FALSE ("Save recipe")
      w127 = sgl[] [] ("FI array")
      w126 = TRUE ("Auto Optimzation")
      w116 = T44."Enabled" ("Disabled")
      w258 = FALSE ("Auto pause")
      w113 = u32 0 ("FIB slice #")
      w117 = FALSE ("Off")
      n84 = local write "Delta Z array"(w127) -> ()
      n85 = local write "Delta X sum array"(w127) -> ()
      n86 = local write "Delta Y sum array"(w127) -> ()
      n87 = local write "Delta image array"(w127) -> ()
      n88 = local write "Milling Z voltage array"(w127) -> ()
      n89 = local write "Re-engage Delta X array"(w127) -> ()
      n90 = local write "Re-engage Delta Y array"(w127) -> ()
      n91 = local write "Re-engage X shift array"(w127) -> ()
      n92 = local write "Re-engage Y shift array"(w127) -> ()
      n93 = local write "Temp array"(w127) -> ()
      n94 = local write "Faraday Cup array"(w127) -> ()
      n95 = local write "SEM Specimen I array"(w127) -> ()
      n96 = local write "Beam Dump 1 array"(w127) -> ()
      n97 = local write "Beam Dump 2 array"(w127) -> ()
      n98 = local write "Milling I array"(w127) -> ()
      n99 = local write "Focus index array"(w127) -> ()
      n100 = local write "Delta X array"(w127) -> ()
      n101 = local write "Delta Y array"(w127) -> ()
      n102 = local write "Specimen I array"(w127) -> ()
      n103 = To Variant(anything=T20 {"Actual scan rate"=0.0, "X resolution with rampdown"=0, "Actual sample rate"=0.0, "Fetch backlog"=0.0, "Total scan points"=0, "Frame rate (/s)"=0} ("type")) -> (Variant=w340:variant)
      n104 = local read "SEM Status"() -> (w329:T12)
      n105 = shared-variable ".\\Zeiss Library.lvlib\\Realtime Imaging Info"(w340) -> ()  [unwired: 1 in, 1 out]
      n106 = To Variant(anything=w329) -> (Variant=w328:variant)
      n107 = Unbundle By Name("Hardware Configuration") -> ("SEM X coil"=w283:refnum<k15>, "SEM Y coil"=w334:refnum<k15>, "FIB X coil"=w335:tag, "FIB Y coil"=w336:tag, "FIB Detector"=w337:tag, "SEM Detectors"=w281:refnum<k15>, "Det min (V)"=w331:dbl, "Det max (V)"=w332:dbl, "Eanable COM"=w276:bool, "COM port"=w333:refnum<visa-resource-name>, "FIB Beam blank"=w321:tag, "FIB Ext Scan"=w318:tag, "Det. FIB-NI auto switch"=w322:tag, "Post #1up"=w275:tag, "Post #1down"=w299:tag, "Post #2up"=w298:tag, "Post #2down"=w274:tag, "Machine Type"=w311:u8, "Machine ID"=w182:string, "Logging Device"=w266:tag)
      "COM port" <- w333
      "Machine Type" <- w311
      "Log Device" <- w266
      "Post #1up" <- w275
      "Post #1down" <- w299
      "Post #2up" <- w298
      "Post #2down" <- w274
      n108 = shared-variable ".\\Zeiss Library.lvlib\\SEMInfo"(w328) -> ()  [unwired: 2 out]
      n109 = local write "Temp high limit array"(w127) -> ()
      n110 = local write "Temp low limit array"(w127) -> ()
      n111 = local write "Specimen I high limit array"(w127) -> ()
      n112 = local write "Specimen I low limit array"(w127) -> ()
      n113 = local write "SEM Specimen I high limit array"(w127) -> ()
      n114 = local write "SEM Specimen I low limit array"(w127) -> ()
      n115 = local write "FI low limit array"(w127) -> ()
      n116 = local write "Faraday Cup high limit array"(w127) -> ()
      n117 = local write "Faraday Cup low limit array"(w127) -> ()
      n118 = local write "Image Tabs"(T37."All" ("Image Tabs")) -> ()
      n119 = local write "Stig Options"(enum16{"Defaut", "Stig X", "Stig Y"}."Defaut" ("Stig Options")) -> ()
      n120 = local write "Log time array"(w149) -> ()
      n121 = local write "Cycle time array"(w149) -> ()
      n122 = local write "Cycle time est offset array"(i16[] [] ("FI array")) -> ()
      n123 = call <instrlib>:"niFgen Initialize.vi"("Resource Name"=w283) -> ("error out"=w284:errorcluster, "Instrument Handle Out"=w294:refnum<k15>)  [unwired: 9 in]
      n124 = call <instrlib>:"niScope Initialize.vi"("resource name"=w281) -> ("instrument handle"=w295:refnum<k15>, "error out"=w290:errorcluster)  [unwired: 13 in]
      n125 = case shown="2" w311 {
        tunnel: [10.0 ("X size (V)") 20.0 ("X size (V)") 16.0 ("X size (V)")] -> w315
        tunnel: [90.0 ("X size (V)") 54.0 ("X size (V)") 90.0 ("X size (V)")] -> w314
        tunnel: [500.0 ("X size (V)") 382.193 ("FIB FOV (um)") 500.0 ("X size (V)")] -> w278
        tunnel: [w605 w621 w639] -> w304
        tunnel: [w607 w621 w639] -> w303
        tunnel: [w607 w621 w638] -> w199
        tunnel: ["Low limit (uA)" ("Label.Text") "Low limit (uA)" ("Label.Text") "Low limit (uA)" ("Label.Text")] -> w242
        tunnel: ["High limit (uA)" ("Label.Text") "High limit (uA)" ("Label.Text") "High limit (uA)" ("Label.Text")] -> w241
        tunnel: ["Faraday" ("Label.Text") " B.D. -\n Spec." ("Label.Text") "Faraday" ("Label.Text")] -> w239
        tunnel: ["Faraday Cup (nA)" ("Label.Text") "B.D. - Spec. (nA)" ("Label.Text") "Faraday Cup (nA)" ("Label.Text")] -> w238
        tunnel: [1.4 ("X size (V)") 1.2 ("X size (V)") 1.38 ("X size (V)")] -> w232
        tunnel: [2.0 ("X size (V)") 1.8 ("X size (V)") 2.0 ("X size (V)")] -> w231
        tunnel: [w605 w619 w639] -> w206
        tunnel: [T45."Page Enabled" ("Page Enabled State") T45."Page Disabled & Grayed" ("Page Enabled State") T45."Page Enabled" ("Page Enabled State")] -> w144
        tunnel: [w607 w621 w639] -> w177
        tunnel: [w605 w619 w638] -> w176
        tunnel: [w607 w619 w639] -> w114
        tunnel: [w605 w619 w638] -> w175
        tunnel: [w607 w619 w639] -> w168
        tunnel: [sgl 6.0 ("Overhead (s)") sgl 7.0 ("Overhead (s)") sgl 5.0 ("Overhead (s)")] -> w167
        frame 0, Default {
          w608 = T44."Enabled" ("Disabled")
          w605 = TRUE ("data")
          w607 = FALSE ("data")
          # "Feiss"
          n126 = property on="Turn on FIB gun" class="Bool (strict)"("DisabledEnum"=w608) -> ()  [unwired: 2 in, 2 out]
          n127 = property on="Request to reheat" class="Bool (strict)"("DisabledEnum"=w608) -> ()  [unwired: 2 in, 2 out]
        }
        frame 1 {
          w619 = FALSE ("data")
          w621 = TRUE ("data")
          # "NVision"
        }
        frame 2 {
          w639 = TRUE ("data")
          w638 = FALSE ("data")
          # "Jeiss"
          n128 = invoke class="_EMApi" method="InitialiseRemoting"(reference="Api") -> (reference out=w665:refnum<k7>, error out=w664:errorcluster, "InitialiseRemoting"=w678:i32)  [unwired: 2 in]
          n129 = call "SmartSEM Remote API set float.vi"("error in"=w664, "vValue"=sgl 0.0, "lpszParam"="DP_FIB_LOCK_MAG", "Api"=w665) -> ("error out"=w660:errorcluster, "Api out"=w661:refnum<k7>)  [unwired: 6 in]
          n130 = call "SmartSEM Remote API set string.vi"("error in"=w660, "vValue"="Polaroid 545" ("lpszParam"), "lpszParam"="DP_USE_REF_MAG", "Api"=w661) -> ("error out"=w656:errorcluster, "Api out"=w657:refnum<k7>)  [unwired: 6 in]
          n131 = Equal To 0?(x=w678) -> (x = 0?=w677:bool)
          n132 = case shown="True" w677 {
            frame False {
            }
            frame True {
              n133 = local write "Status message"("API Initialized" ("Status message")) -> ()
            }
          }
          n134 = call "SmartSEM Remote API set string.vi"("error in"=w656, "vValue"="Undefined" ("lpszParam"), "lpszParam"="DP_FIB_MILL_PROBE", "Api"=w657) -> ("error out"=w645:errorcluster, "Api out"=w644:refnum<k7>)  [unwired: 6 in]
          n135 = call "SmartSEM Remote API get string.vi"("error in"=w645, "lpszParam"="DP_FIB_IMAGE_PROBE", "Api"=w644) -> ("error out"=w636:errorcluster, "data"=w652:string, "Api out"=w637:refnum<k7>)  [unwired: 6 in]
          n136 = local write "FIB Milling Probe"(w652) -> ()
          n137 = call "SmartSEM Remote API get float.vi"("error in"=w636, "lpszParam"="AP_FIB_OBJECTIVE_POTENTIAL", "Api"=w637) -> ("error out"=w634:errorcluster, "vValue"=w632:sgl, "Api out"=w635:refnum<k7>)  [unwired: 6 in]
          n138 = call "SmartSEM Remote API set float.vi"("error in"=w634, "vValue"=sgl 1.0, "lpszParam"="DP_AUTO_HYSTERESIS", "Api"=w635) -> ("error out"=w641:errorcluster, "Api out"=w640:refnum<k7>)  [unwired: 6 in]
          n139 = call "SmartSEM Remote API set float.vi"("error in"=w641, "vValue"=sgl 0.0, "lpszParam"="DP_PANEL_DISABLE", "Api"=w640) -> ("error out"=w647:errorcluster, "Api out"=w670:refnum<k7>)  [unwired: 6 in]
          n140 = call "SmartSEM Remote API set float.vi"("error in"=w647, "vValue"=sgl 0.0, "lpszParam"="DP_JOYSTICK_DISABLE", "Api"=w670) -> ("error out"=w646:errorcluster, "Api out"=w650:refnum<k7>)  [unwired: 6 in]
          n141 = call "SmartSEM Remote API get string.vi"("error in"=w646, "lpszParam"="SV_VERSION", "Api"=w650) -> ("data"=w651:string, "Api out"=w648:refnum<k7>)  [unwired: 6 in, 1 out]
          n142 = Scan From String(format string="V%f", input string=w651) -> (output 1=w668:dbl)  [unwired: 3 in, 3 out]
          n143 = Greater Or Equal?(x=w668, y=6.01) -> (x >= y?=w666:bool)
          n144 = case shown="True" w666 {
            tunnel: w648 -> [_ w689]
            frame False {
            }
            frame True {
              n145 = call "SmartSEM Remote API set float.vi"("vValue"=sgl 1.0, "lpszParam"="DP_FIB_SCAN_ROT", "Api"=w689) -> ()  [unwired: 7 in, 2 out]
            }
          }
          n146 = local write "FIB Milling Objective (V)"(w632) -> ()
        }
      }
      "Overhead (s)" <- w167
      n147 = local write "BD1 high limit array"(w127) -> ()
      n148 = local write "BD1 low limit array"(w127) -> ()
      n149 = local write "BD2 high limit array"(w127) -> ()
      n150 = local write "BD2 low limit array"(w127) -> ()
      n151 = local write "Milling I high limit array"(w127) -> ()
      n152 = local write "Milling I low limit array"(w127) -> ()
      n153 = property class="niScope"(reference=w295, error in=w290) -> (reference out=w291:refnum<k15>, error out=w289:errorcluster, "Maximum Real Time Sample Rate"=w280:dbl)
      n154 = property class="niFgen"(reference=w294, error in=w284) -> (reference out=w286:refnum<k15>, error out=w285:errorcluster, "Sample Rate"=w282:dbl)
      n155 = Bundle By Name(cluster="SEM HW Config", "SEM X coil"=w283, "SEM Y coil"=w334, "Detectors A&B"=w281, "Det min (V)"=w331, "Det max (V)"=w332, "Eanable COM"=w276, "COM port"=w333, "Detector FIB-NI auto switch"=w322, "Machine Type"=w311, "Machine ID"=w182) -> (w296:T9)
      n156 = call "FIB ext scan.vi"("Ext on"=FALSE ("data"), "FIB Ext Scan"=w318) -> ()  [unwired: 9 in, 1 out]
      n157 = call <instrlib>:"niFgen Abort Generation.vi"("error in (no error)"=w285, "Instrument Handle"=w286) -> ("error out"=w288:errorcluster, "Instrument Handle Out"=w287:refnum<k15>)  [unwired: 8 in]
      n158 = call <instrlib>:"niFgen Close.vi"("error in (no error)"=w288, "Instrument Handle"=w287) -> ()  [unwired: 9 in, 1 out]
      n159 = Bundle By Name(cluster="FIB HW Config", "FIB X coil"=w335, "FIB Y coil"=w336, "Beam blank"=w321, "FIB Ext Scan"=w318, "Detector"=w337, "Post #1up"=w275, "Post #1down"=w299, "Post #2up"=w298, "Post #2down"=w274) -> (w339:T23)
      n160 = local read "Api"() -> (w124:refnum<k7>)
      n161 = call <instrlib>:"niScope Abort.vi"("instrument handle"=w291, "error in"=w289) -> ("instrument handle out"=w293:refnum<k15>, "error out"=w292:errorcluster)  [unwired: 12 in]
      n162 = call "FIB beam blank.vi"("Api"=w124, "Beam blanked"=TRUE, "lines"=w321) -> ()  [unwired: 2 in, 1 out]
      n163 = call <instrlib>:"niScope Close.vi"("instrument handle"=w293, "error in"=w292) -> ()  [unwired: 13 in, 1 out]
      n164 = local write "SEM HW Config"(w296) -> ()
      n165 = case shown="False" w276 {
        tunnel: [T44."Disabled and Grayed Out" ("Disabled") T44."Enabled" ("Disabled")] -> w277
        frame False {
        }
        frame True {
        }
      }
      n166 = local write "FIB HW Config"(w339) -> ()
      n167 = local write "Auto Optimzation"(w126) -> ()
      n168 = local write "3D image paused armed"(w126) -> ()
      n169 = local write "FIB emission limit warning armed"(w126) -> ()
      n170 = local write "SW error warning armed"(w126) -> ()
      n171 = local write "Focus index warning armed"(w126) -> ()
      n172 = local write "Re-engage warning armed"(w126) -> ()
      n173 = local write "FIB emission limit warning active"(w117) -> ()
      n174 = local write "SW error warning active"(w117) -> ()
      n175 = local write "SEM shutter failed active"(w117) -> ()
      n176 = local write "Focus index recovery active"(w117) -> ()
      n177 = local write "Focus index warning active"(w117) -> ()
      n178 = local write "Temperature recovery active"(w117) -> ()
      n179 = local write "Temperature warning active"(w117) -> ()
      n180 = local read "SEM Status"() -> (w325:T12)
      n181 = Bundle By Name(cluster=w325, "AO SampClk.MaxRate"=w282, "AI SampClk.MaxRate"=w280) -> (w326:T12)
